vi "Layout - Parse VI for Subpanel Control Reference.vi"(8 "error in (no error)":errorcluster, 10 "SubPanel Label":string, 11 "VI in":refnum<vi>) -> (0 "error out":errorcluster, 3 "SubPanel Ref":refnum<vi>)   [LabVIEW 2022 SP3, in "UI Manager.lvlib"]
doc: "Parses the <b>VI in</b> for a subpanel labelled <b>SubPanel Label</b> and returns the reference to it.\n\n____\nHAMPEL SOFTWARE ENGINEERING v2.6.0 (2023-12-19 10:54)"
uses:
  UI Manager.lvlib
  <vilib>/Utility/traverseref.llb/TRef TravTarget.ctl
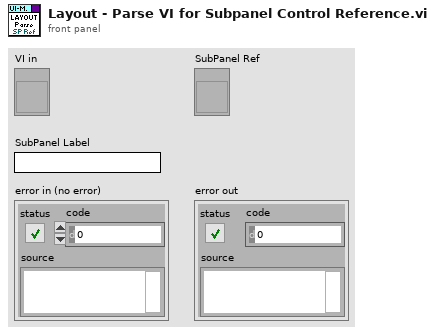
[diagram p1: front panel]
types:
  T1 = typedef "TRef TravTarget.ctl" = enum16{"FP", "BD", "Other"}
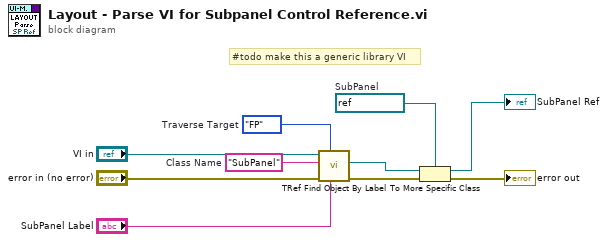
[diagram p0: block diagram]
diagram:
  w5 = refnum<vi> refnum  # SubPanel
  w2 = TRef_TravTarget."FP"  # Traverse Target
  w1 = "SubPanel"  # Class Name
  # "#todo make this a generic library VI"
  n1 = call <vilib>:"TRef Find Object By Label.vi"("Label"="SubPanel Label", "Traverse Target"=w2, "error in (no error)"="error in (no error)", "Class Name"=w1, "VI Ref"="VI in") -> ("error out"=w4:errorcluster, "Found Obj Ref"=w3:refnum<vi>)  [unwired: 3 in, 2 out]
  n2 = To More Specific Class(target class=w5, reference=w3, error in=w4) -> (specific class reference=→"SubPanel Ref":refnum<vi>, error out=→"error out":errorcluster)
